vi "Distance From Pixels.vi"(11 "Width":dbl) -> (3 "Distance":dbl)   [LabVIEW 2012]
panel:
  in  "x 2":dbl=0.5
  in  "x":dbl=0.5
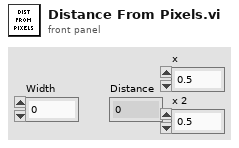
[diagram p1: front panel]
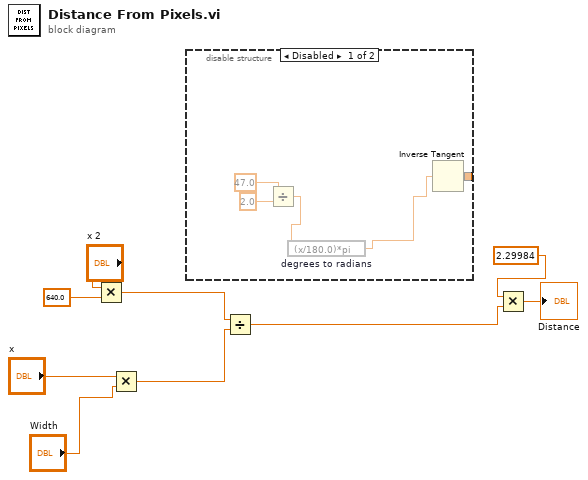
[diagram p0: block diagram]
diagram:
  n1 = Multiply(x="x 2", y=640.0) -> (x*y=w4:dbl)
  n2 = Multiply(x="x", y="Width") -> (x*y=w8:dbl)
  n3 = disable-structure shown="Disabled" {
    disable-tunnel: [w10 _] -> _
    frame Disabled {
      n4 = Divide(x=47.0, y=2.0) -> (x/y=w14:dbl)
      n5 = expression code="(x/180.0)*pi" "degrees to radians"(w14) -> (w11:dbl)
      n6 = Inverse Tangent(1:w11) -> (0:w10:dbl)
    }
    frame Enabled {
    }
  }
  n7 = Divide(x=w4, y=w8) -> (x/y=w5:dbl)
  n8 = Multiply(x=2.29984, y=w5) -> (x*y=→"Distance":dbl)
